vi "BrowerComponent_New.vi"(0 "reference in":refnum<class "BrowerComponent.lvclass">, 1 "Object name":string, 5 "error in (no error)":errorcluster, 6 "CreateMethod(Create or look up existing)":T1(ring)) -> (14 "reference out":refnum<class "BrowerComponent.lvclass">, 15 "NewObjectCreated":bool, 16 "DVRRefOut":refnum<data-value>, 19 "error out":errorcluster)   [LabVIEW 2015, in "BrowerComponent.lvclass"]
uses:
  BrowerComponent.lvclass
  protected/ObjectAttributes.ctl
  BrowerComponent.lvclass/BrowerComponent.ctl
panel:
  in  "DVRRef(Hidden)":refnum<data-value>
  in  "Data":T2
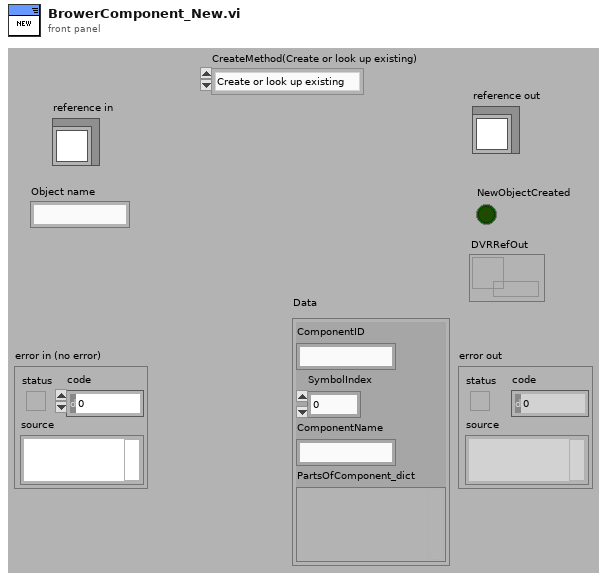
[diagram p1: front panel]
types:
  T1 = enum16{"Create or look up existing", "Look up existing"}
  T2 = typedef "BrowerComponent.lvclass/ObjectAttributes.ctl" = cluster{"ComponentID":string, "SymbolIndex":i32, "ComponentName":string, "PartsOfComponent_dict":variant}
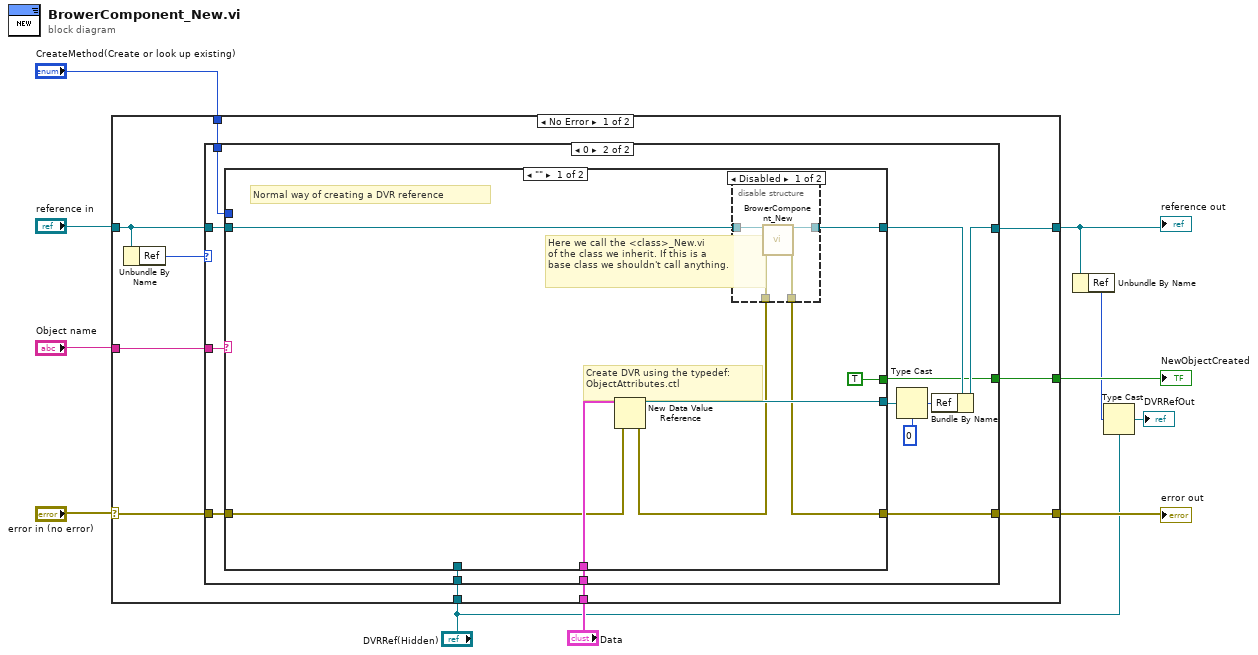
[diagram p0: block diagram]
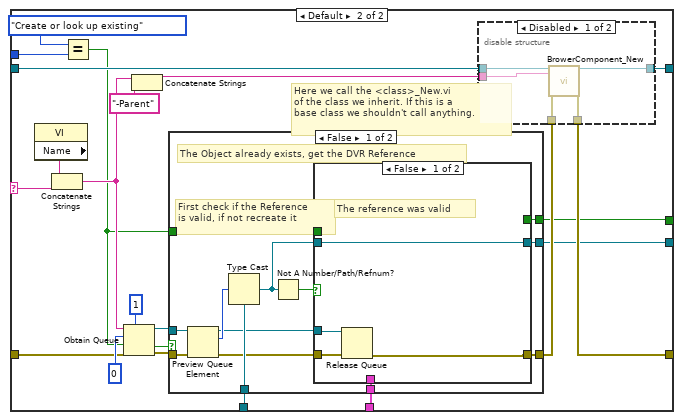
[diagram p4: hidden frame]
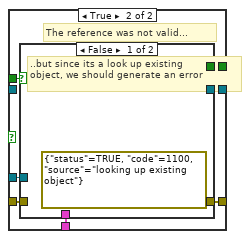
[diagram p5: hidden frame]
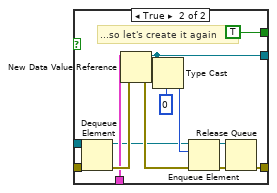
[diagram p6: hidden frame]
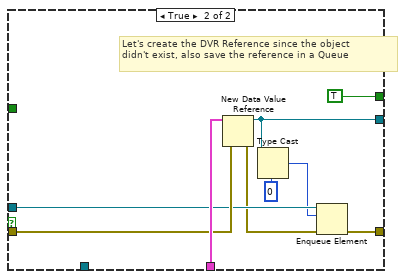
[diagram p7: hidden frame]
diagram:
  n1 = case shown="No Error" "error in (no error)" {
    selector: "error in (no error)" -> [w21 w128]
    tunnel: [w18 w128] -> w7
    tunnel: "CreateMethod(Create or look up existing)" -> [w19 _]
    tunnel: "Object name" -> [w20 _]
    tunnel: "Data" -> [w17 _]
    tunnel: "DVRRef(Hidden)" -> [w16 _]
    tunnel: "reference in" -> [w15 w127]
    tunnel: [w14 w127] -> w3
    tunnel: [w13 _] -> w5
    frame No Error {
      n2 = Unbundle By Name(w15) -> ("Ref"=w12:u32)
      n3 = case shown="0" w12 {
        tunnel: w21 -> [w23 w27]
        tunnel: w20 -> [_ w36]
        tunnel: w19 -> [_ w35]
        tunnel: [w23 w34] -> w18
        tunnel: w17 -> [_ w33]
        tunnel: w15 -> [w22 w31]
        tunnel: [w22 w32] -> w14
        tunnel: w16 -> [_ w29]
        tunnel: [_ w28] -> w13
        frame Default {
          # "The DVR reference has already been created, from this child class's <Child>_New.vi"
        }
        frame 0 {
          n4 = case shown="\"\"" w36 {
            selector: w36 -> [_ w64]
            tunnel: [w38 w61] -> w34
            tunnel: w35 -> [_ w71]
            tunnel: w33 -> [w44 w55]
            tunnel: [w42 w53] -> w25
            tunnel: w31 -> [w41 w70]
            tunnel: [w40 w69] -> w30
            tunnel: w29 -> [_ w56]
            tunnel: [TRUE ("created new?") w52] -> w28
            tunnel: w27 -> [w43 w62]
            frame "" {
              # "Create DVR using the typedef:\nObjectAttributes.ctl"
              # "Here we call the <class>_New.vi\nof the class we inherit. If this is a\nbase class we shouldn't call anything."
              # "Normal way of creating a DVR reference"
              n5 = New Data Value Reference(data value=w44, error in=w43) -> (data value reference=w42:refnum<data-value>, error out=w39:errorcluster)
              n6 = disable-structure shown="Disabled" {
                disable-tunnel: w41 -> [w48 w50]
                disable-tunnel: [w47 w50] -> w40
                disable-tunnel: w39 -> [w46 w49]
                disable-tunnel: [w45 w49] -> w38
                frame Disabled {
                  n7 = call "BrowerComponent_New.vi"("reference in"=w48, "error in (no error)"=w46) -> ("reference out"=w47:refnum<class "BrowerComponent.lvclass">, "error out"=w45:errorcluster)  [unwired: 14 in, 2 out]
                }
                frame Enabled {
                }
              }
            }
            frame Default {
              # "Here we call the <class>_New.vi\nof the class we inherit. If this is a\nbase class we shouldn't call anything."
              n8 = property class="VI"() -> ("Name"=w65:string)  [unwired: 2 in, 2 out]
              n9 = Concatenate Strings(w65, w64) -> (w63:string)
              n10 = Equal?(x=T1."Create or look up existing", y=w71) -> (x = y?=w57:bool)
              n11 = Obtain Queue(max queue size (-1, unlimited)=1, name (unnamed)=w63, element data type=u32 0 ("DataRef"), create if not found? (T)=w57, error in (no error)=w62) -> (queue out=w58:refnum<queue>, created new?=w59:bool, error out=w60:errorcluster)
              n12 = Concatenate Strings(w63, "-Parent" ("string")) -> (w66:string)
              n13 = case shown="False" w59 {
                tunnel: w60 -> [w84 w118]
                tunnel: w55 -> [w75 w119]
                tunnel: w58 -> [w85 w117]
                tunnel: [w79 w114] -> w54
                tunnel: [w77 w113] -> w53
                tunnel: w56 -> [w82 _]
                tunnel: [w74 TRUE] -> w52
                tunnel: w57 -> [w73 _]
                frame False {
                  # "First check if the Reference\nis valid, if not recreate it"
                  # "The Object already exists, get the DVR Reference"
                  n14 = Preview Queue Element(queue=w85, error in (no error)=w84) -> (queue out=w76:refnum<queue>, element=w83:u32, error out=w81:errorcluster)  [unwired: 1 in, 1 out]
                  n15 = Type Cast(type=w82, x=w83) -> (*(type *) &x=w78:refnum<data-value>)
                  n16 = Not A Number/Path/Refnum?(number/path/refnum=w78) -> (NaN/Path/Refnum?=w80:bool)
                  n17 = case shown="False" w80 {
                    tunnel: w81 -> [w87 w95]
                    tunnel: [w86 w92] -> w79
                    tunnel: w78 -> [w89 _]
                    tunnel: [w89 w93] -> w77
                    tunnel: w76 -> [w88 w96]
                    tunnel: w75 -> [_ w94]
                    tunnel: [_ w91] -> w74
                    tunnel: w73 -> [_ w90]
                    frame False {
                      # "The reference was valid"
                      n18 = Release Queue(queue=w88, error in (no error)=w87) -> (error out=w86:errorcluster)  [unwired: 1 in, 2 out]
                    }
                    frame True {
                      # "The reference was not valid..."
                      n19 = case shown="False" w90 {
                        tunnel: w96 -> [_ w110]
                        tunnel: w95 -> [_ w109]
                        tunnel: w94 -> [_ w105]
                        tunnel: [_ w102] -> w93
                        tunnel: [errorcluster {"status"=TRUE, "code"=1100, "source"="looking up existing object"} ("error out") w98] -> w92
                        tunnel: [_ TRUE] -> w91
                        frame False {
                          # "..but since its a look up existing\nobject, we should generate an error"
                        }
                        frame True {
                          # "...so let's create it again"
                          n20 = Dequeue Element(queue=w110, error in (no error)=w109) -> (queue out=w103:refnum<queue>, error out=w106:errorcluster)  [unwired: 1 in, 2 out]
                          n21 = New Data Value Reference(data value=w105, error in=w106) -> (data value reference=w102:refnum<data-value>, error out=w104:errorcluster)
                          n22 = Type Cast(type=u32 0 ("ObjectQueue"), x=w102) -> (*(type *) &x=w107:u32)
                          n23 = Enqueue Element(queue=w103, element=w107, error in (no error)=w104) -> (queue out=w99:refnum<queue>, error out=w100:errorcluster)  [unwired: 1 in, 1 out]
                          n24 = Release Queue(queue=w99, error in (no error)=w100) -> (error out=w98:errorcluster)  [unwired: 1 in, 2 out]
                        }
                      }
                    }
                  }
                }
                frame True {
                  # "Let's create the DVR Reference since the object\ndidn't exist, also save the reference in a Queue"
                  n25 = New Data Value Reference(data value=w119, error in=w118) -> (data value reference=w113:refnum<data-value>, error out=w115:errorcluster)
                  n26 = Type Cast(type=u32 0 ("ObjectQueue"), x=w113) -> (*(type *) &x=w112:u32)
                  n27 = Enqueue Element(queue=w117, element=w112, error in (no error)=w115) -> (error out=w114:errorcluster)  [unwired: 1 in, 2 out]
                }
              }
              n28 = disable-structure shown="Disabled" {
                disable-tunnel: w70 -> [w124 w126]
                disable-tunnel: [w123 w126] -> w69
                disable-tunnel: w66 -> [w122 _]
                disable-tunnel: w54 -> [w121 w125]
                disable-tunnel: [w120 w125] -> w61
                frame Disabled {
                  n29 = call "BrowerComponent_New.vi"("reference in"=w124, "Object name"=w122, "error in (no error)"=w121) -> ("reference out"=w123:refnum<class "BrowerComponent.lvclass">, "error out"=w120:errorcluster)  [unwired: 13 in, 2 out]
                }
                frame Enabled {
                }
              }
            }
          }
          n30 = Type Cast(type=u32 0 ("DataRef"), x=w25) -> (*(type *) &x=w24:u32)
          n31 = Bundle By Name(cluster=w30, "Ref"=w24) -> (w32:refnum<class "BrowerComponent.lvclass">)
        }
      }
    }
    frame Error {
    }
  }
  "error out" <- w7
  "reference out" <- w3
  "NewObjectCreated" <- w5
  n32 = Unbundle By Name(w3) -> ("Ref"=w4:u32)
  n33 = Type Cast(type="DVRRef(Hidden)", x=w4) -> (*(type *) &x=→"DVRRefOut":refnum<data-value>)
